vi "IsFrameOK.vi"(9 "inputdata new":string, 11 "inputdata old":string) -> (1 "frame ok":bool, 3 "outputdata":string)   [LabVIEW 2012]
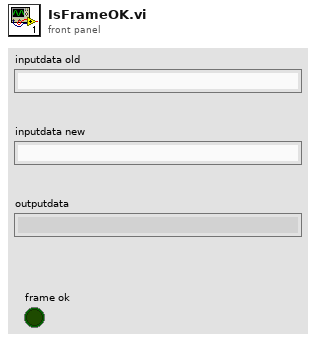
[diagram p1: front panel]
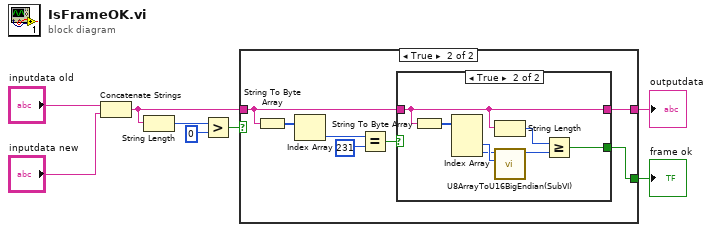
[diagram p0: block diagram]
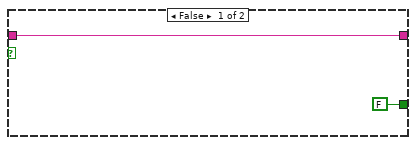
[diagram p2: hidden frame]
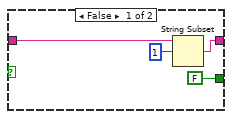
[diagram p3: hidden frame]
diagram:
  n1 = Concatenate Strings("inputdata old", "inputdata new") -> (w1:string)
  n2 = String Length(string=w1) -> (length=w8:i32)
  n3 = Greater?(x=w8, y=0) -> (0:w6:bool)
  n4 = case shown="True" w6 {
    tunnel: w1 -> [w10 w13]
    tunnel: [w10 w12] -> w5
    tunnel: [FALSE w11] -> w4
    frame False {
    }
    frame True {
      n5 = String To Byte Array(string=w13) -> (unsigned byte array=w16:u8[])
      n6 = Index Array(array=w16) -> (element=w15:u8)  [unwired: 1 in]
      n7 = Equal?(x=w15, y=u8 231) -> (x = y?=w14:bool)
      n8 = case shown="True" w14 {
        tunnel: w13 -> [w21 w22]
        tunnel: [w19 w22] -> w12
        tunnel: [FALSE w23] -> w11
        frame False {
          n9 = String Subset(string=w21, offset (0)=1) -> (substring=w19:string)  [unwired: 1 in]
        }
        frame True {
          n10 = String To Byte Array(string=w22) -> (unsigned byte array=w28:u8[])
          n11 = Index Array(array=w28) -> (element #2=w27:u8, element #3=w26:u8)  [unwired: 3 in, 1 out]
          n12 = String Length(string=w22) -> (length=w25:i32)
          n13 = call "U8ArrayToU16BigEndian(SubVI).vi"("Numeric 7"=w27, "Numeric 6"=w26) -> ("Numeric 9"=w24:u16)  [unwired: 9 in]
          n14 = Greater Or Equal?(x=w25, y=w24) -> (x >= y?=w23:bool)
        }
      }
    }
  }
  "outputdata" <- w5
  "frame ok" <- w4
